vi "AutoRocketCargo.vi"(10 "RightSideOfField?":bool, 11 "Coordinates":dbl[](array[numeric])) -> ()   [LabVIEW 2018]
uses:
  Globals.vi
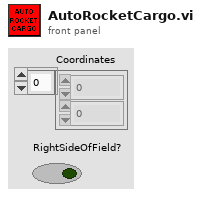
[diagram p1: front panel]
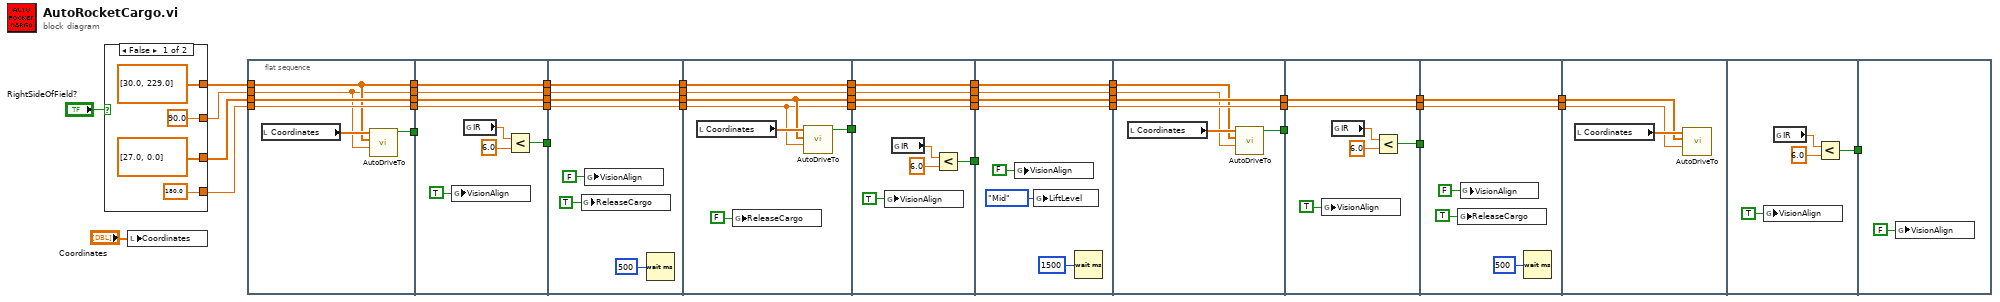
[diagram p0: block diagram]
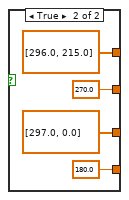
[diagram p2: hidden frame]
diagram:
  n1 = case shown="False" "RightSideOfField?" {
    tunnel: [dbl[] [27.0, 0.0] dbl[] [297.0, 0.0]] -> w40
    tunnel: [90.0 270.0] -> w41
    tunnel: [dbl[] [30.0, 229.0] dbl[] [296.0, 215.0]] -> w42
    tunnel: [180.0 180.0] -> w39
    frame False {
    }
    frame True {
    }
  }
  n2 = local write "Coordinates"("Coordinates") -> ()
  n3 = flat-sequence {
    tunnel: [w57] -> w37
    tunnel: w42 -> [w53]
    tunnel: w41 -> [w52]
    tunnel: w40 -> [w56]
    tunnel: w39 -> [w55]
    tunnel: [w56] -> w36
    tunnel: [w55] -> w35
    tunnel: [w53] -> w34
    tunnel: [w52] -> w33
    tunnel: [w62] -> w9
    tunnel: w37 -> [_]
    tunnel: w36 -> [w61]
    tunnel: w35 -> [w60]
    tunnel: [w61] -> w8
    tunnel: [w60] -> w7
    tunnel: [w59] -> w6
    tunnel: w34 -> [w59]
    tunnel: w33 -> [w58]
    tunnel: [w58] -> w5
    tunnel: w9 -> [_]
    tunnel: w8 -> [w72]
    tunnel: [w72] -> w4
    tunnel: w7 -> [w71]
    tunnel: [w71] -> w3
    tunnel: w6 -> [w70]
    tunnel: [w70] -> w2
    tunnel: w5 -> [w69]
    tunnel: [w69] -> w1
    tunnel: w4 -> [w75]
    tunnel: w3 -> [w74]
    tunnel: [w78] -> w20
    tunnel: [w77] -> w19
    tunnel: w2 -> [w77]
    tunnel: w1 -> [w76]
    tunnel: [w76] -> w17
    tunnel: [w75] -> w15
    tunnel: [w74] -> w13
    tunnel: w20 -> [_]
    tunnel: w19 -> [w87]
    tunnel: [w87] -> w18
    tunnel: w17 -> [w86]
    tunnel: [w86] -> w16
    tunnel: w15 -> [w85]
    tunnel: [w85] -> w14
    tunnel: w13 -> [w84]
    tunnel: [w84] -> w12
    tunnel: [w81] -> w11
    tunnel: [w94] -> w32
    tunnel: w18 -> [w94]
    tunnel: [w93] -> w31
    tunnel: w16 -> [w93]
    tunnel: [w92] -> w30
    tunnel: w14 -> [w92]
    tunnel: [w91] -> w29
    tunnel: w12 -> [w91]
    tunnel: w11 -> [_]
    tunnel: w32 -> [w97]
    tunnel: w31 -> [w96]
    tunnel: w30 -> [w100]
    tunnel: w29 -> [w99]
    tunnel: [w100] -> w28
    tunnel: [w99] -> w27
    tunnel: [w95] -> w26
    tunnel: w28 -> [w106]
    tunnel: w27 -> [w105]
    tunnel: [w106] -> w25
    tunnel: [w105] -> w24
    tunnel: [w101] -> w23
    tunnel: w26 -> [_]
    tunnel: w25 -> [w111]
    tunnel: w24 -> [w110]
    tunnel: w23 -> [_]
    tunnel: [w111] -> w22
    tunnel: [w110] -> w21
    tunnel: w22 -> [w113]
    tunnel: w21 -> [w112]
    tunnel: [w115] -> w10
    tunnel: w10 -> [_]
    frame #0 {
      n4 = local read "Coordinates"() -> (w54:dbl[])
      n5 = call "AutoDriveTo.vi"("EndAngle"=w52, "EndCoordinates"=w53, "Coordinates"=w54) -> ("ThereYet?"=w57:bool)  [unwired: 8 in]
    }
    frame #1 {
      n6 = global write "Globals.vi" "VisionAlign"(TRUE ("VisionAlign")) -> ()
      n7 = global read "Globals.vi" "IR"() -> (w64:dbl)
      n8 = Less?(x=w64, y=6.0) -> (x < y?=w62:bool)
    }
    frame #2 {
      n9 = global write "Globals.vi" "ReleaseCargo"(TRUE ("ReleaseCargo")) -> ()
      n10 = global write "Globals.vi" "VisionAlign"(FALSE ("VisionAlign")) -> ()
      n11 = Wait (ms)(milliseconds to wait=u32 500) -> ()  [unwired: 1 out]
    }
    frame #3 {
      n12 = local read "Coordinates"() -> (w79:dbl[])
      n13 = global write "Globals.vi" "ReleaseCargo"(FALSE ("ReleaseCargo")) -> ()
      n14 = call "AutoDriveTo.vi"("EndAngle"=w74, "EndCoordinates"=w75, "Coordinates"=w79) -> ("ThereYet?"=w78:bool)  [unwired: 8 in]
    }
    frame #4 {
      n15 = global write "Globals.vi" "VisionAlign"(TRUE ("VisionAlign")) -> ()
      n16 = global read "Globals.vi" "IR"() -> (w83:dbl)
      n17 = Less?(x=w83, y=6.0) -> (x < y?=w81:bool)
    }
    frame #5 {
      n18 = global write "Globals.vi" "VisionAlign"(FALSE ("VisionAlign")) -> ()
      n19 = global write "Globals.vi" "LiftLevel"(enum16{"Low", "Mid", "High"}."Mid" ("LiftLevel")) -> ()
      n20 = Wait (ms)(milliseconds to wait=u32 1500) -> ()  [unwired: 1 out]
    }
    frame #6 {
      n21 = local read "Coordinates"() -> (w98:dbl[])
      n22 = call "AutoDriveTo.vi"("EndAngle"=w96, "EndCoordinates"=w97, "Coordinates"=w98) -> ("ThereYet?"=w95:bool)  [unwired: 8 in]
    }
    frame #7 {
      n23 = global write "Globals.vi" "VisionAlign"(TRUE ("VisionAlign")) -> ()
      n24 = global read "Globals.vi" "IR"() -> (w103:dbl)
      n25 = Less?(x=w103, y=6.0) -> (x < y?=w101:bool)
    }
    frame #8 {
      n26 = global write "Globals.vi" "ReleaseCargo"(TRUE ("ReleaseHatch")) -> ()
      n27 = global write "Globals.vi" "VisionAlign"(FALSE ("VisionAlign")) -> ()
      n28 = Wait (ms)(milliseconds to wait=u32 500) -> ()  [unwired: 1 out]
    }
    frame #9 {
      n29 = local read "Coordinates"() -> (w114:dbl[])
      n30 = call "AutoDriveTo.vi"("EndAngle"=w112, "EndCoordinates"=w113, "Coordinates"=w114) -> ()  [unwired: 8 in, 1 out]
    }
    frame #10 {
      n31 = global write "Globals.vi" "VisionAlign"(TRUE ("VisionAlign")) -> ()
      n32 = global read "Globals.vi" "IR"() -> (w117:dbl)
      n33 = Less?(x=w117, y=6.0) -> (x < y?=w115:bool)
    }
    frame #11 {
      n34 = global write "Globals.vi" "VisionAlign"(FALSE ("VisionAlign")) -> ()
    }
  }
